vi "MQTT_PingReq.vi"(8 "error in (no error)":errorcluster, 11 "connection ID":refnum<k5>) -> (0 "error out":errorcluster, 2 "PingReq Message":u8[](array[numeric]) format="%x", 3 "connection ID out":refnum<k5>)   [LabVIEW 2018, in "MQTT_Functions.lvlib"]
uses:
  MQTT_Functions.lvlib
  Controls/MessageType.ctl
  Controls/Retain_Flag.ctl
  Controls/QoS.ctl
  Controls/DUP_Flag.ctl
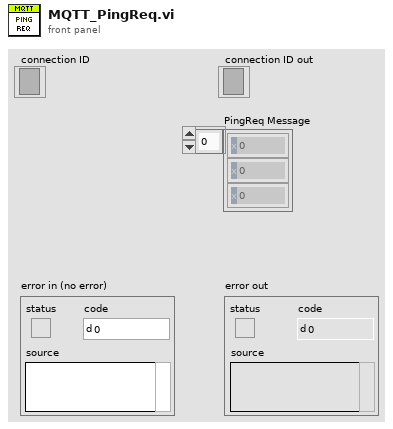
[diagram p1: front panel]
types:
  T1 = typedef "MQTT_Functions.lvlib/DUP_Flag.ctl" = bool
  T2 = typedef "MQTT_Functions.lvlib/QoS.ctl" = enum8{"At most once", "At least once", "Exactly once", "Reserved"}
  T3 = typedef "MQTT_Functions.lvlib/Retain_Flag.ctl" = bool
  T4 = typedef "MQTT_Functions.lvlib/MessageType.ctl" = enum32{"Reserved", "CONNECT", "CONNACK", "PUBLISH", "PUBACK", "PUBREC", "PUBREL", "PUBCOMP", "SUBSCRIBE", "SUBACK", "UNSUBSCRIBE", "UNSUBACK", "PINGREQ", "PINGRESP", "DISCONNECT", "Reserved2"}
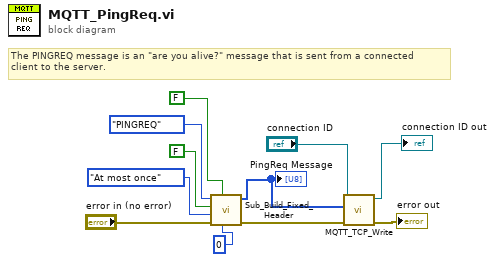
[diagram p0: block diagram]
diagram:
  # "The PINGREQ message is an \"are you alive?\" message that is sent from a connected\nclient to the server."
  n1 = call "Sub_Build_Fixed_Header.vi"("Remaining Length"=u32 0, "Retain"=T3 FALSE, "error in (no error)"="error in (no error)", "QoS"=QoS."At most once", "DUP"=T1 FALSE, "MessageType"=MessageType."PINGREQ") -> ("error out"=w5:errorcluster, "Fixed Header"=w1:u8[])  [unwired: 4 in]
  "PingReq Message" <- w1
  n2 = call "MQTT_TCP_Write.vi"("error in (no error)"=w5, "data in"=w1, "connection ID"="connection ID") -> ("error out"=→"error out":errorcluster, "connection ID out"=→"connection ID out":refnum<k5>)  [unwired: 6 in, 1 out]
